vi "SA40144D.20210728 2D in vacuum.vi"() -> ()   [LabVIEW 2020]
uses:
  <vilib>/Analysis/baseanly.llb/Mean (DBL).vi
  <userlib>/_OpenG.lib/file/file.llb/Build Path - Traditional__ogtk.vi
  <userlib>/LevyLab/LV to ITX/Data/Data.lvclass
  <userlib>/LevyLab/XY Utilities/xy_utilities.lvlib
  <vilib>/Analysis/NI_AALBase.lvlib
panel:
  in  "Tab Control":enum32{"Page 1", "Page 2"}(tab)
  out "G2T vs t - X channel":T1(graph)
  out "G4T vs t - X channel":T1(graph)
  out "Temp vs t":T1(graph)
  out "Arrhenius":T1(graph)
  out "Y6 - dV":T1(graph)
  out "Y5 - I-":T1(graph)
  out "X5 - I-":T1(graph)
  out "X6 - dV":T1(graph)
  in  "Temps to keep (Lifespan)":i32=26
  out "E_a":dbl[](array[numeric])
  in  "Temps to keep (Arrhenius fit)":i32=26
  in  "Source Voltage":dbl=0.1
  in  "Init Temp":i32=275
  in  "Temp Step":i32=5
  in  "Final Temp":i32=400
  in  "Data File":path=path "G:/My Drive/ansom/Data/PPMS 2/SA40144D.20210728/00 - BG in vacuum/SA40144D.20210728.275K.dat"
  in  "Trimming":i32=400
  in  "Update":bool
  in  "OK":bool
  out "error out":errorcluster
  in  "error in (no error)":errorcluster
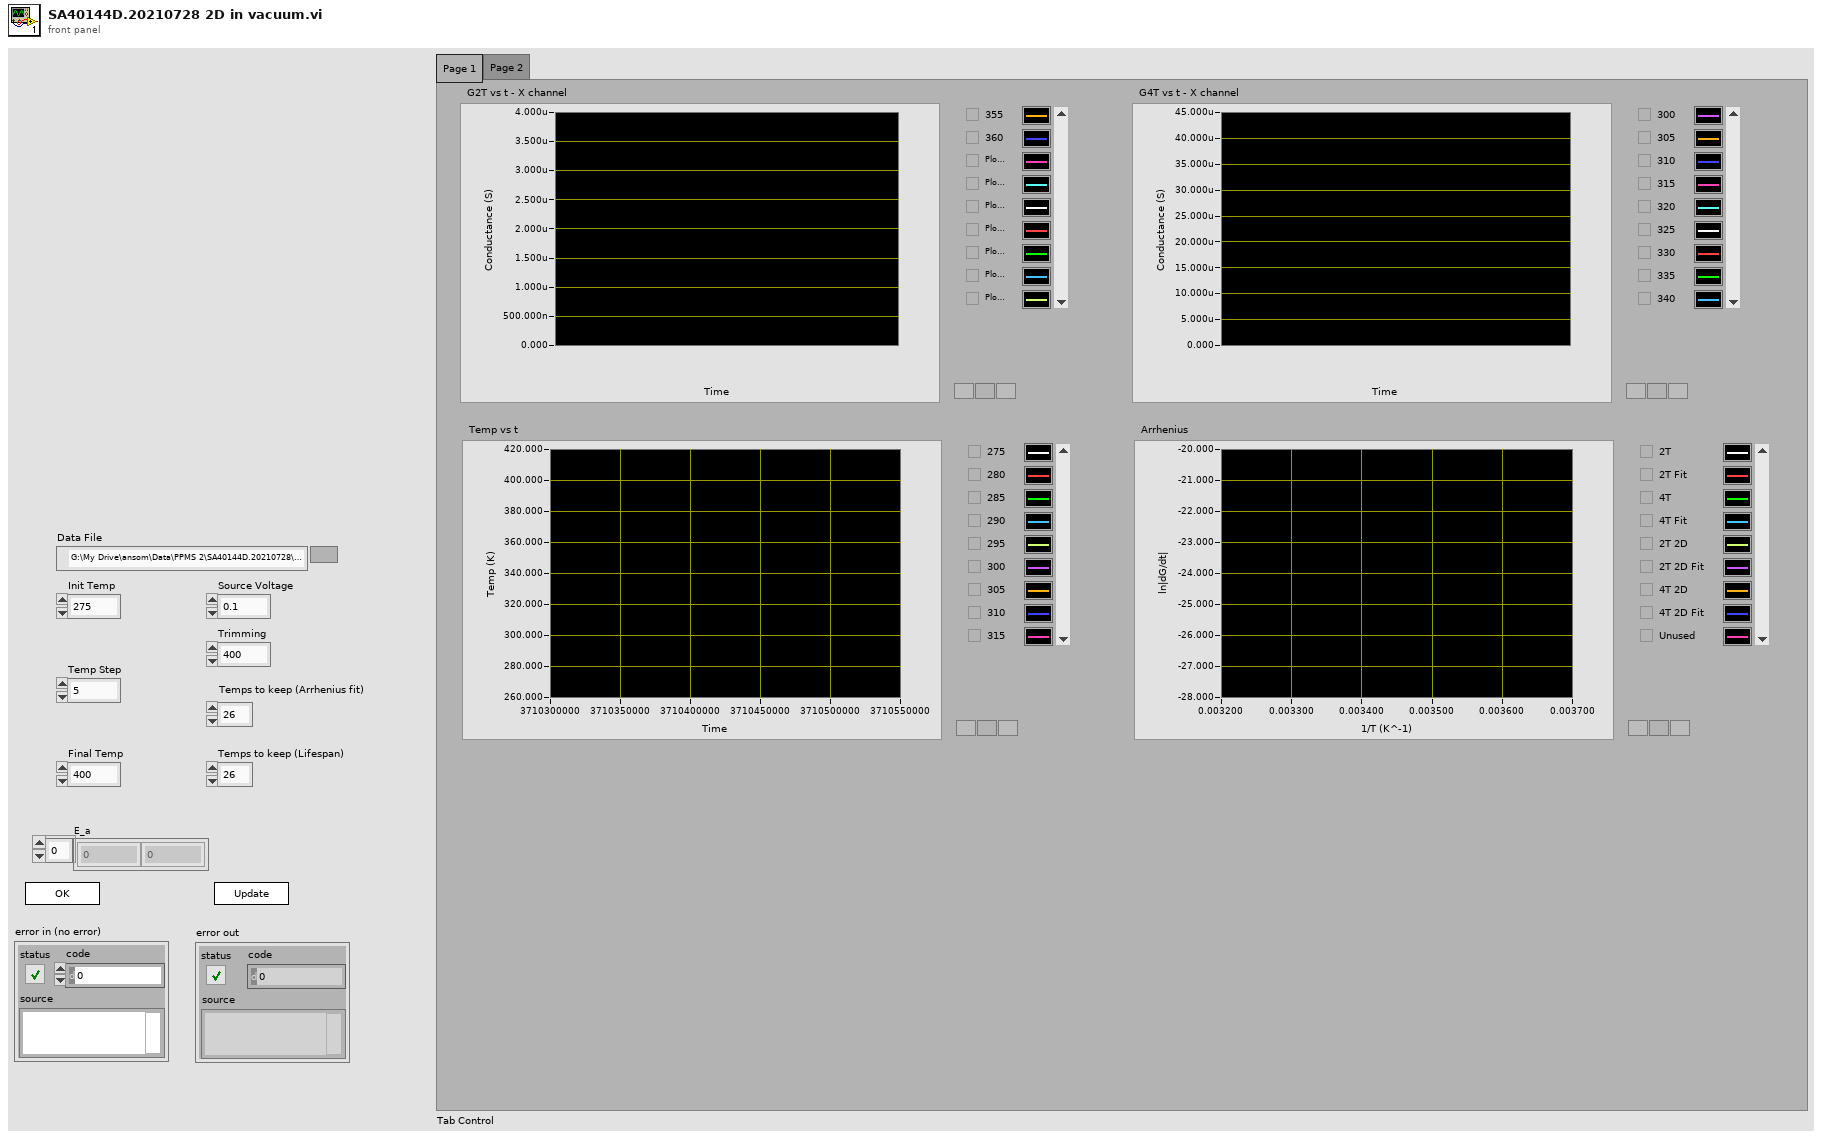
[diagram p1: front panel]
types:
  T1 = cluster{"Data":dbl[], "Best Exponential Fit":dbl[]}[]
  T2 = enum32{"Invalid", "Standard", "Closed", "Hidden", "Minimized", "Maximized"}
  T3 = enum32{"invalid app kind", "Development System", "Run Time System", "Student Edition", "Embedded LabVIEW", "Evaluation", "Custom"}
  T4 = cluster{"Core":cluster{"Current VI Reference":refnum<vi>, "Close Panel on Exit?":bool}, "G2T 1D":cluster{dbl[], dbl[]}[], "G4T 1D":cluster{dbl[], dbl[]}[], "X11":cluster{dbl[], dbl[]}[], "X15":cluster{dbl[], dbl[]}[], "Temp":cluster{dbl[], dbl[]}[], "G2T BG":cluster{dbl[], dbl[]}[], "Source Voltage":dbl, "Final Temp":i32, "Init Temp":i32, "Temp Step":i32, "Data File":path, "Trimming":i32}
  T5 = cluster{"Current VI Reference":refnum<vi>, "Close Panel on Exit?":bool}
  T6 = typedef "Data.lvclass/Dictionary--cluster.ctl" = cluster{"key":string, "value":variant}
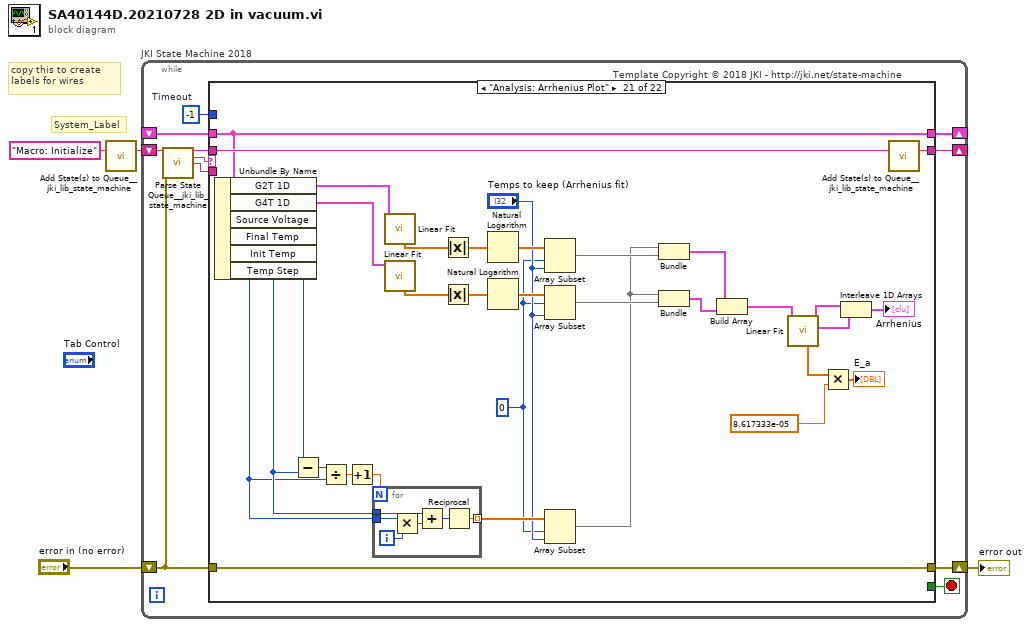
[diagram p0: block diagram]
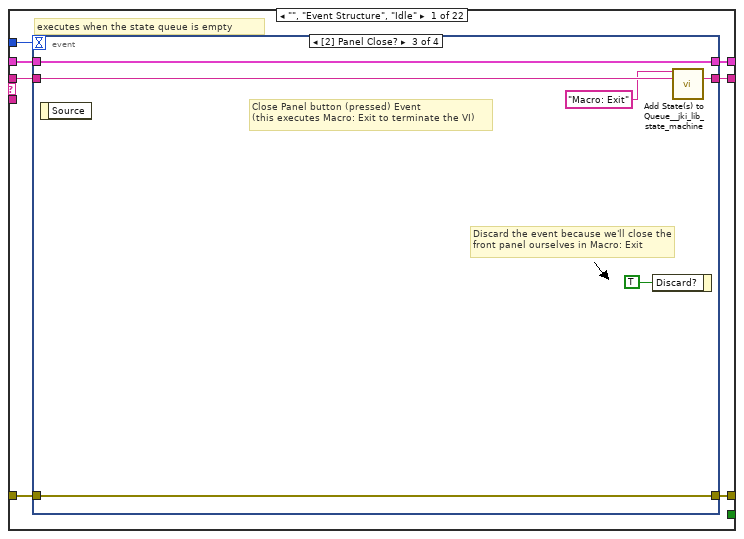
[diagram p2: hidden frame]
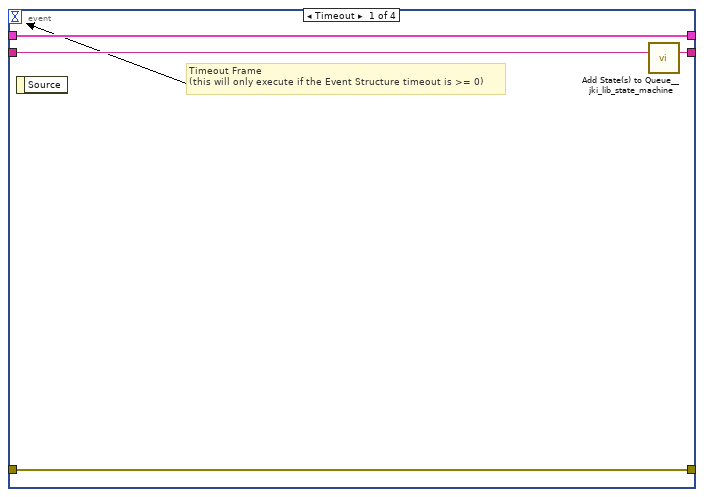
[diagram p3: hidden frame]
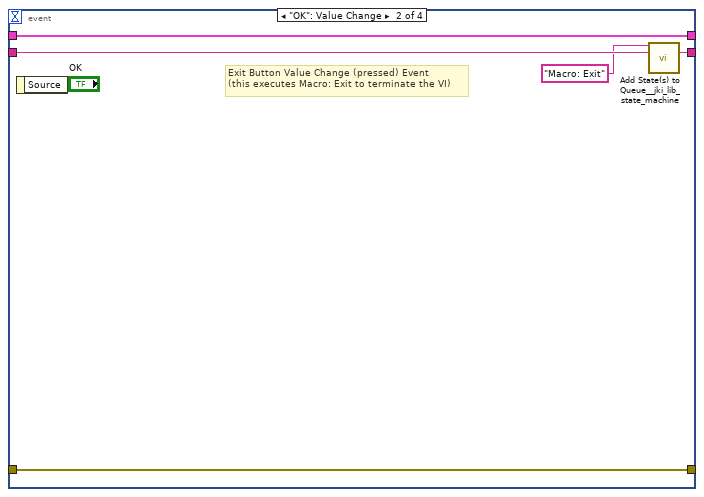
[diagram p4: hidden frame]
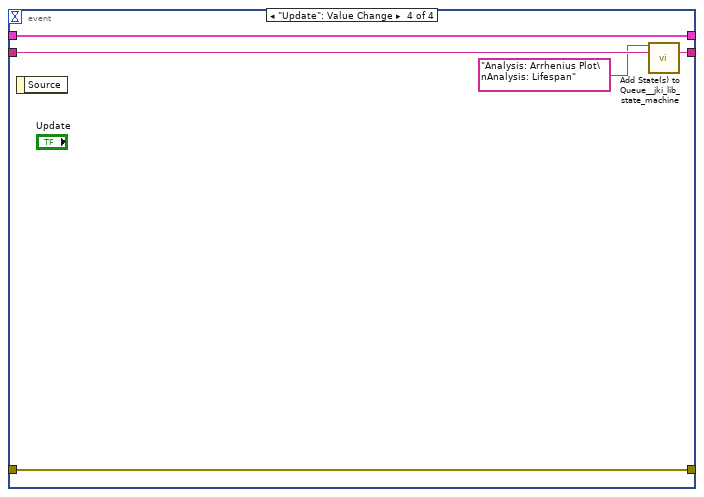
[diagram p5: hidden frame]
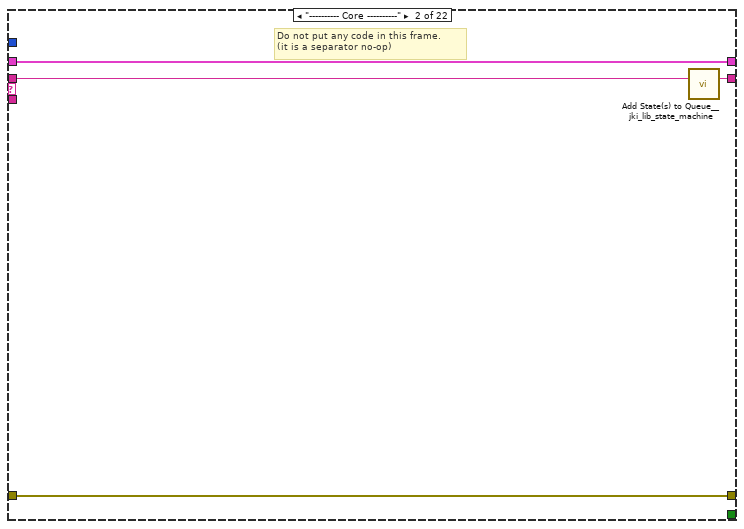
[diagram p6: hidden frame]
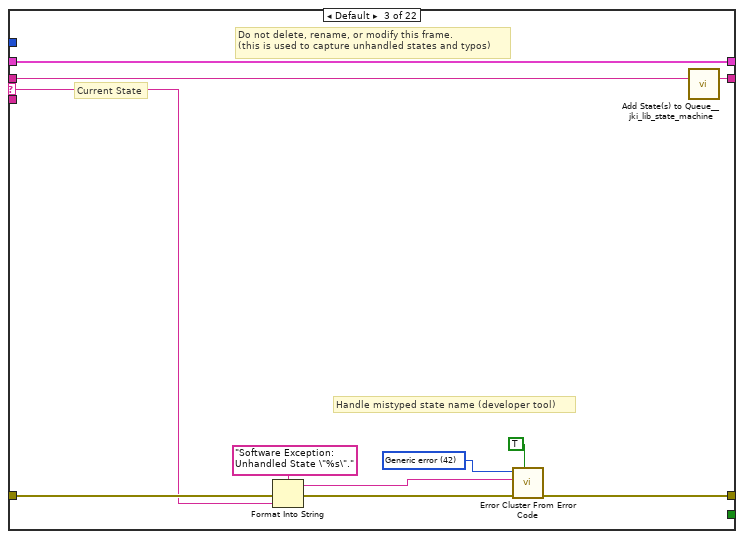
[diagram p7: hidden frame]
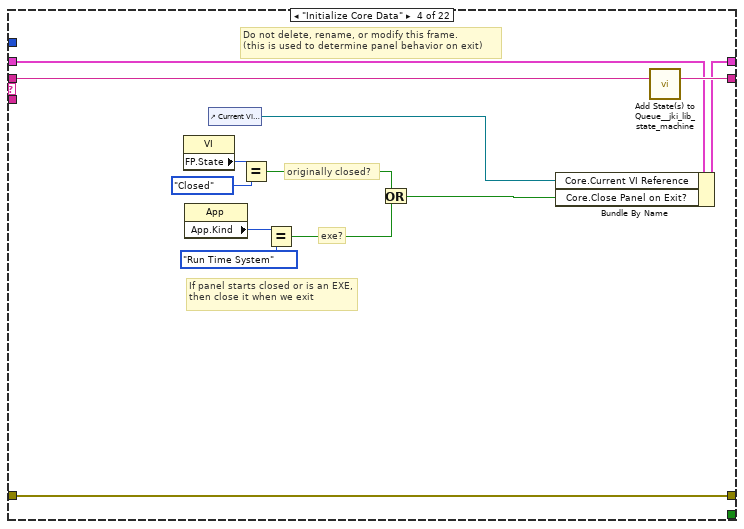
[diagram p8: hidden frame]
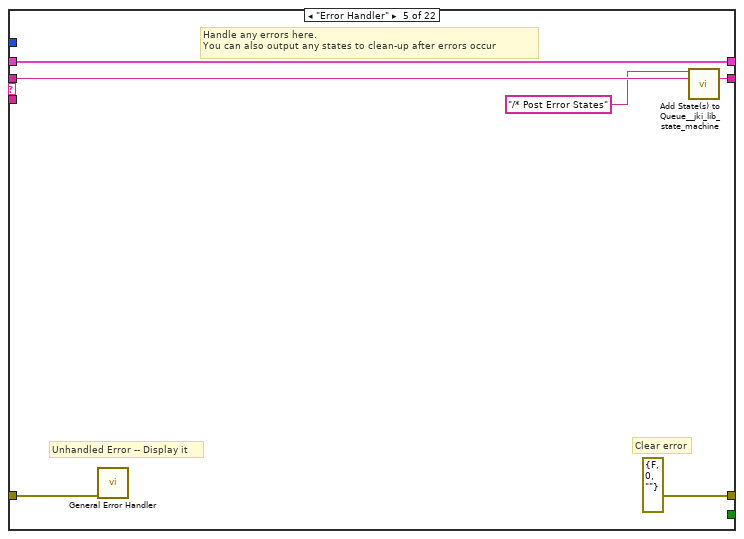
[diagram p9: hidden frame]
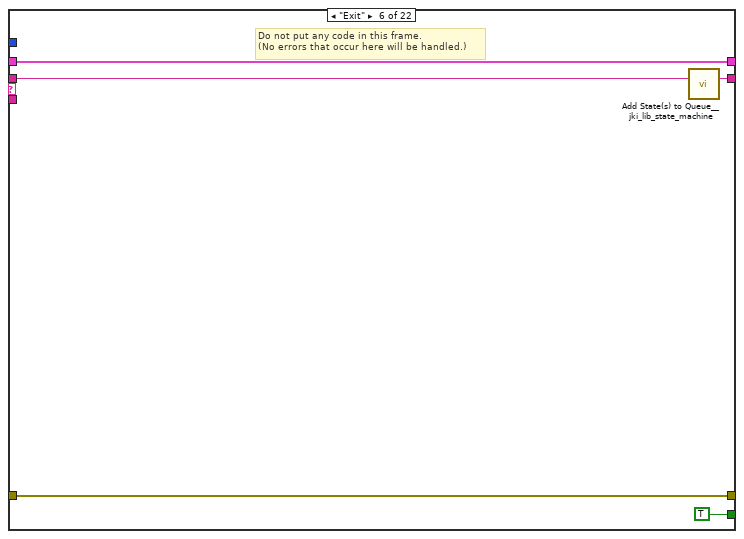
[diagram p10: hidden frame]
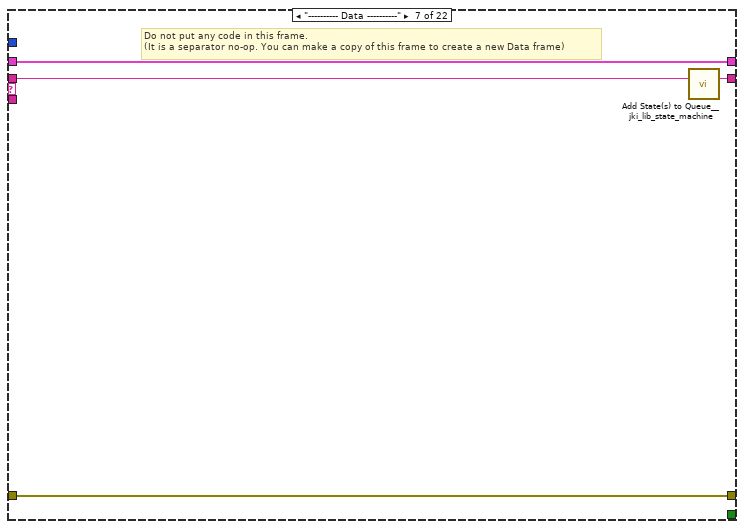
[diagram p11: hidden frame]
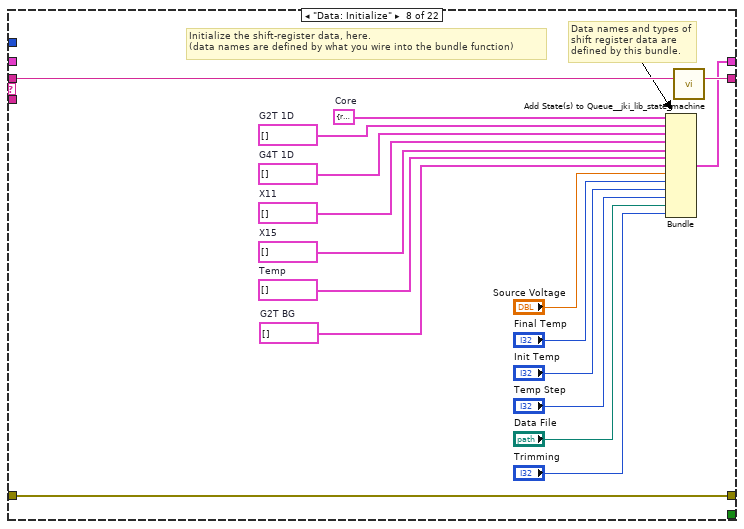
[diagram p12: hidden frame]
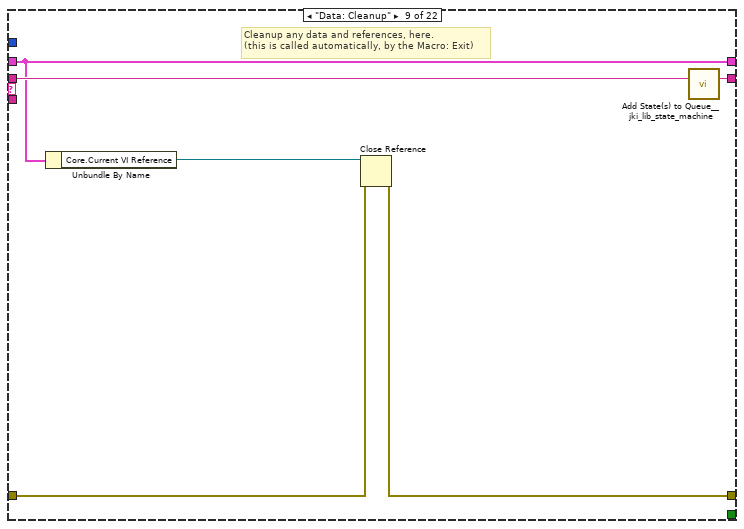
[diagram p13: hidden frame]
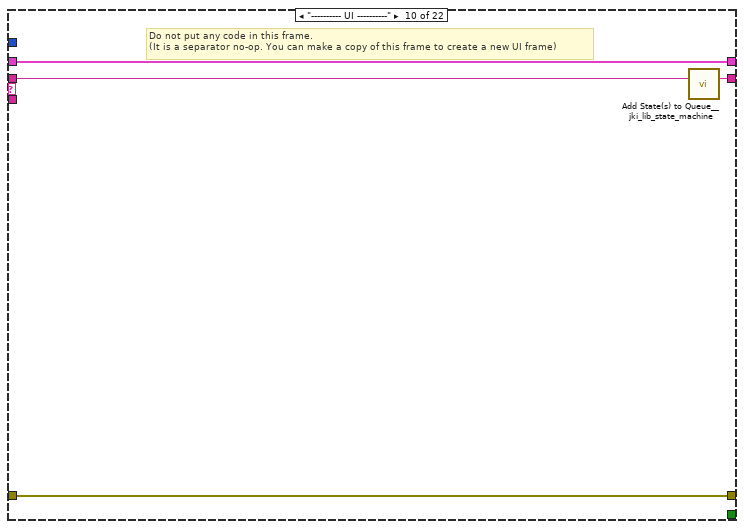
[diagram p14: hidden frame]
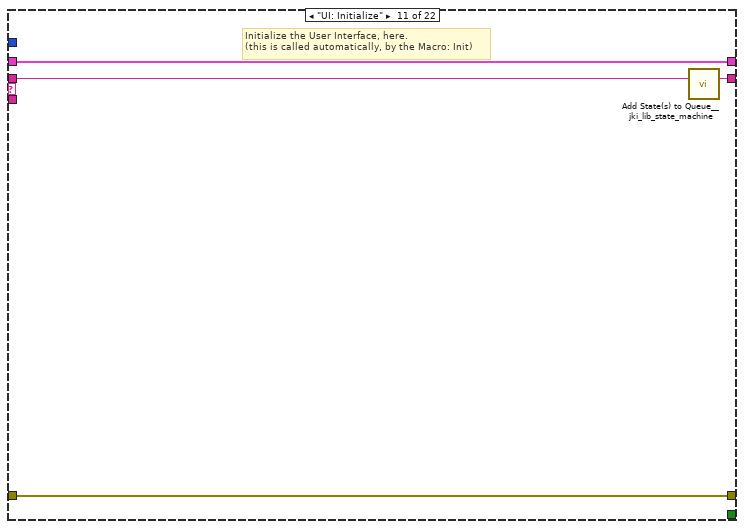
[diagram p15: hidden frame]
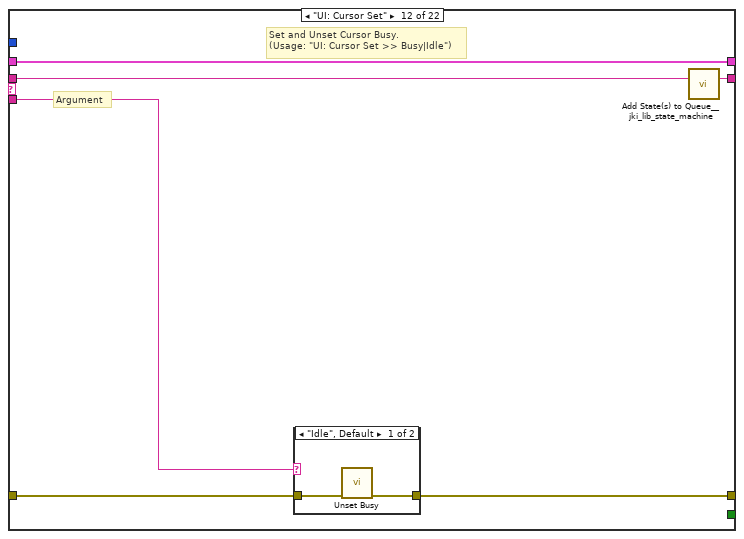
[diagram p16: hidden frame]
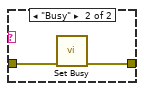
[diagram p17: hidden frame]
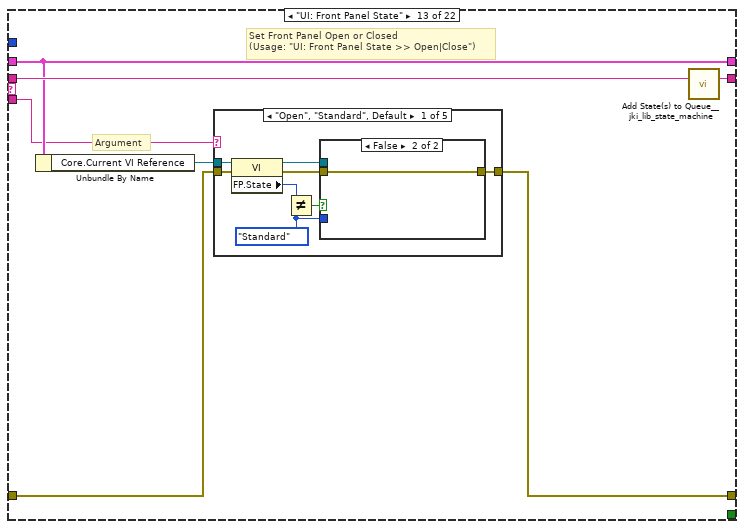
[diagram p18: hidden frame]
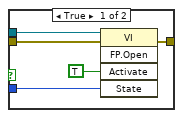
[diagram p19: hidden frame]
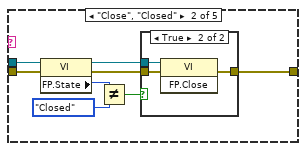
[diagram p20: hidden frame]
diagram:
  # "copy this to create labels for wires"
  # "System_Label"
  n1 = call <vilib>:"Add State(s) to Queue__jki_lib_state_machine.vi"("State(s) in (\"\")"="Macro: Initialize") -> ("States Out"=w4:string)  [unwired: 14 in]
  n2 = while "JKI State Machine 2018" {
    shift-right: [w8] -> _
    shift-left: _ -> [w7]
    shift-right: [w11] -> w1
    shift-left: "error in (no error)" -> [w5]
    shift-right: [w10] -> _
    shift-left: w4 -> [w12]
    stop <- w9 stop-if-true
    w6 = -1  # Timeout
    # "Template Copyright © 2018 JKI - http://jki.net/state-machine"
    n3 = call <vilib>:"Parse State Queue__jki_lib_state_machine.vi"("State Queue"=w12, "Error In (no error)"=w5) -> ("Remaining States"=w14:string, "Current State"=w15:string, "Arguments"=w13:string)  [unwired: 11 in]
    n4 = case shown="\"Analysis: Arrhenius Plot\"" w15 {
      selector: w15 -> [_ _ w47 _ _ _ _ _ _ _ _ _ _ _ _ _ _ _ _ _ _ _]
      tunnel: w14 -> [w22 w46 w51 w70 w76 w81 w85 w102 w108 w112 w116 w122 w133 w202 w207 w217 w221 w238 w295 w339 w372 w410]
      tunnel: w13 -> [_ _ _ _ _ _ _ _ _ _ _ w117 w127 _ _ _ _ _ _ _ _ _]
      tunnel: w7 -> [w20 w43 w49 w63 w73 w79 w82 _ w103 w109 w114 w120 w129 w199 w204 w214 w218 w232 w289 w336 w369 w396]
      tunnel: [w19 w44 w53 w67 errorcluster {"status"=FALSE, "code"=0, "source"=""} ("error out") w78 w83 w99 w104 w110 w113 w118 w130 w200 w205 w215 w219 w234 w291 w337 w370 w408] -> w11
      tunnel: w5 -> [w18 w44 w52 w67 w72 w78 w83 w99 w105 w110 w113 w119 w131 w200 w205 w215 w219 w234 w291 w337 w370 w408]
      tunnel: [w21 w45 w50 w69 w75 w80 w84 w101 w107 w111 w115 w121 w132 w201 w206 w216 w220 w237 w294 w338 w371 w409] -> w10
      tunnel: [_ _ _ _ _ TRUE _ _ _ _ _ _ _ _ _ _ _ _ _ _ _ _] -> w9
      tunnel: [w17 w43 w49 w68 w73 w79 w82 w100 w103 w109 w114 w120 w129 w199 w204 w214 w218 w233 w290 w336 w369 w396] -> w8
      tunnel: w6 -> [w16 _ _ _ _ _ _ _ _ _ _ _ _ _ _ _ _ _ _ _ _ _]
      frame "", "Event Structure", "Idle" {
        # "executes when the state queue is empty"
        n5 = event shown="[2] Panel Close?" {
          selector: _ -> [_ _ _ _]
          dyn-events: _ -> [_ _ _ _]
          timeout: w16 -> [_ _ _ _]
          tunnel: w22 -> [w26 w31 w37 w41]
          tunnel: [w25 w30 w36 w40] -> w21
          tunnel: w20 -> [w23 w28 w34 w42]
          tunnel: [w24 w29 w35 w38] -> w19
          tunnel: w18 -> [w24 w29 w35 w38]
          tunnel: [w23 w28 w34 w42] -> w17
          event Timeout {
            # "Timeout Frame\n(this will only execute if the Event Structure timeout is >= 0)"
            n6 = event-data() -> ()  [unwired: 1 in, 1 out]
            n7 = call <vilib>:"Add State(s) to Queue__jki_lib_state_machine.vi"("State(s) in (\"\")"=w26) -> ("States Out"=w25:string)  [unwired: 14 in]
          }
          event "OK": Value Change {
            # "Exit Button Value Change (pressed) Event\n(this executes Macro: Exit to terminate the VI)"
            n8 = event-data() -> ()  [unwired: 1 in, 1 out]
            n9 = call <vilib>:"Add State(s) to Queue__jki_lib_state_machine.vi"("State(s) in Front (\"\")"="Macro: Exit", "State(s) in (\"\")"=w31) -> ("States Out"=w30:string)  [unwired: 13 in]
          }
          event Panel Close? {
            # "Discard the event because we'll close the front panel ourselves in Macro: Exit"
            # "Close Panel button (pressed) Event\n(this executes Macro: Exit to terminate the VI)"
            n10 = event-data() -> ()  [unwired: 1 in, 1 out]
            n11 = event-data("Discard?"=TRUE) -> ()  [unwired: 1 in, 1 out]
            n12 = call <vilib>:"Add State(s) to Queue__jki_lib_state_machine.vi"("State(s) in Front (\"\")"="Macro: Exit", "State(s) in (\"\")"=w37) -> ("States Out"=w36:string)  [unwired: 13 in]
          }
          event "Update": Value Change {
            n13 = event-data() -> ()  [unwired: 1 in, 1 out]
            n14 = call <vilib>:"Add State(s) to Queue__jki_lib_state_machine.vi"("State(s) in Front (\"\")"="Analysis: Arrhenius Plot\nAnalysis: Lifespan" ("State(s) in Front (\"\")"), "State(s) in (\"\")"=w41) -> ("States Out"=w40:string)  [unwired: 13 in]
          }
        }
      }
      frame "---------- Core ----------" {
        # "Do not put any code in this frame.\n(it is a separator no-op)"
        n15 = call <vilib>:"Add State(s) to Queue__jki_lib_state_machine.vi"("State(s) in (\"\")"=w46) -> ("States Out"=w45:string)  [unwired: 14 in]
      }
      frame Default {
        w56 = 42 items=["No error", "Argument error", "Memory is full", "Out of zone", "End of file", "File already open", "Generic file I/O error", "File not found", "File permission error", "Disk is full", "Duplicate path", "Too many files open", "System feature not enabled", "Resource file not found", "Cannot add resource", "Resource not found", "Image not found", "Image memory error", "Pen does not exist", "Config type invalid", "Config token not found", "Config parse error", "Config memory error", "Bad external code format", "Bad external code offset", "External code not present", "Null window", "Destroy window error", "Null menu", "Print aborted", "Bad print record", "Print driver error", "Windows error during printing", "Memory error during printing", "Print dialog error", "Generic print error", "Invalid device refnum", "Device not found", "Device parameter error", "Device unit error", "Cannot open device", "Device call aborted", "Generic error", "Cancelled by user", "Object ID too low", "Object ID too high", "Object not in heap", "Unknown heap", "Unknown object (invalid DefProc)", "Unknown object (DefProc not in table)", "Message out of range", "Invalid (null) method", "Unknown message", "Manager call not supported", "Bad address", "Network operation in progress", "Network operation timed out", "Connection is busy", "Network attribute not supported", "Network error", "Address in use", "System out of memory", "Connection aborted", "Connection refused", "Not connected", "Already connected", "Connection closed", "Initialization error (interapplication manager)", "Bad occurrence", "Wait on unbound occurrence handler", "Occurrence queue overflow", "Datalog type conflict", "Unused", "Unrecognized type (interapplication manager)", "Memory corrupt", "Failed to make temporary DLL", "Old CIN version", "Drag socket not found", "Failed to load drop-object", "Failed to register OLE object", "Failed to release OLE object", "Format specifier type mismatch", "Unknown format specifier", "Too few format specifiers", "Too many format specifiers", "Scan failed", "Newer CIN version", "Error converting to variant", "Runtime menu error", "Password tampered", "Variant attribute not found", "Incompatible variant data type", "Event data is not available", "Event Store is not present", "Occurrence is not found", "Event Queue is not created", "Event info is not available", "Refnum passed is NULL", "Error retrieving Class GUID", "Error retrieving CoClass GUID", "Error retrieving TypeLib GUID.", "Bad built application magic bytes.", "Specific driver is different from the specific driver associated with the Logical Name.", "There is no session opened to the class driver.", "Max Error", "MAX - Error with config objects", "MAX - Error loading configuration", "MAX - Group not supported"]
        # "Current State"
        # "Do not delete, rename, or modify this frame.\n(this is used to capture unhandled states and typos)"
        # "Handle mistyped state name (developer tool)"
        n16 = Format Into String(format string="Software Exception: Unhandled State \"%s\"." ("message"), error in=w52, w47) -> (resulting string=w55:string, error out=w54:errorcluster)  [unwired: 1 in]
        n17 = call <vilib>:"Error Cluster From Error Code.vi"("show call chain? (False)"=TRUE, "error in (no error)"=w54, "error message (\"\")"=w55, "error code (0)"=w56) -> ("error out"=w53:errorcluster)  [unwired: 5 in]
        n18 = call <vilib>:"Add State(s) to Queue__jki_lib_state_machine.vi"("State(s) in (\"\")"=w51) -> ("States Out"=w50:string)  [unwired: 14 in]
      }
      frame "Initialize Core Data" {
        # "Do not delete, rename, or modify this frame.\n(this is used to determine panel behavior on exit)"
        # "originally closed?"
        # "exe?"
        # "If panel starts closed or is an EXE, then close it when we exit"
        n19 = property class="VI"() -> ("FP.State"=w60:T2)  [unwired: 2 in, 2 out]
        n20 = property class="App"() -> ("App.Kind"=w66:T3)  [unwired: 2 in, 2 out]
        n21 = control-ref of="Current VI Reference"() -> (w61:refnum<vi>)
        n22 = Equal?(x=w60, y=T2."Closed" ("Front Panel Window:State")) -> (x = y?=w58:bool)
        n23 = Equal?(x=w66, y=T3."Run Time System" ("Application:Kind")) -> (x = y?=w64:bool)
        n24 = Or(x=w58, y=w64) -> (x .or. y?=w62:bool)
        n25 = Bundle By Name(cluster=w63, "Core.Current VI Reference"=w61, "Core.Close Panel on Exit?"=w62) -> (w68:T4)
        n26 = call <vilib>:"Add State(s) to Queue__jki_lib_state_machine.vi"("State(s) in (\"\")"=w70) -> ("States Out"=w69:string)  [unwired: 14 in]
      }
      frame "Error Handler" {
        # "Unhandled Error -- Display it"
        # "Handle any errors here.\nYou can also output any states to clean-up after errors occur"
        # "Clear error"
        n27 = call <vilib>:"General Error Handler.vi"("error in (no error)"=w72) -> ()  [unwired: 10 in, 5 out]
        n28 = call <vilib>:"Add State(s) to Queue__jki_lib_state_machine.vi"("State(s) in Front (\"\")"="/* Post Error States", "State(s) in (\"\")"=w76) -> ("States Out"=w75:string)  [unwired: 13 in]
      }
      frame "Exit" {
        # "Do not put any code in this frame.\n(No errors that occur here will be handled.)"
        n29 = call <vilib>:"Add State(s) to Queue__jki_lib_state_machine.vi"("State(s) in (\"\")"=w81) -> ("States Out"=w80:string)  [unwired: 14 in]
      }
      frame "---------- Data ----------" {
        # "Do not put any code in this frame.\n(It is a separator no-op. You can make a copy of this frame to create a new Data frame)"
        n30 = call <vilib>:"Add State(s) to Queue__jki_lib_state_machine.vi"("State(s) in (\"\")"=w85) -> ("States Out"=w84:string)  [unwired: 14 in]
      }
      frame "Data: Initialize" {
        w86 = cluster{dbl[], dbl[]}[] []  # G2T BG
        w87 = cluster{dbl[], dbl[]}[] []  # Temp
        w96 = cluster{dbl[], dbl[]}[] []  # X15
        w95 = cluster{dbl[], dbl[]}[] []  # X11
        w94 = cluster{dbl[], dbl[]}[] []  # G4T 1D
        w93 = cluster{dbl[], dbl[]}[] []  # G2T 1D
        w98 = T5 {"Current VI Reference"=refnum, "Close Panel on Exit?"=FALSE}  # Core
        # "Data names and types of shift register data are defined by this bundle."
        # "Initialize the shift-register data, here.\n(data names are defined by what you wire into the bundle function)"
        n31 = Bundle("Core"=w98, "G2T 1D"=w93, "G4T 1D"=w94, "X11"=w95, "X15"=w96, "Temp"=w87, "G2T BG"=w86, "Source Voltage"="Source Voltage", "Final Temp"="Final Temp", "Init Temp"="Init Temp", "Temp Step"="Temp Step", "Data File"="Data File", "Trimming"="Trimming") -> (w100:T4)  [unwired: 1 in]
        n32 = call <vilib>:"Add State(s) to Queue__jki_lib_state_machine.vi"("State(s) in (\"\")"=w102) -> ("States Out"=w101:string)  [unwired: 14 in]
      }
      frame "Data: Cleanup" {
        # "Cleanup any data and references, here.\n(this is called automatically, by the Macro: Exit)"
        n33 = Unbundle By Name(w103) -> ("Core.Current VI Reference"=w106:refnum<vi>)
        n34 = Close Reference(reference=w106, error in (no error)=w105) -> (error out=w104:errorcluster)
        n35 = call <vilib>:"Add State(s) to Queue__jki_lib_state_machine.vi"("State(s) in (\"\")"=w108) -> ("States Out"=w107:string)  [unwired: 14 in]
      }
      frame "---------- UI ----------" {
        # "Do not put any code in this frame.\n(It is a separator no-op. You can make a copy of this frame to create a new UI frame)"
        n36 = call <vilib>:"Add State(s) to Queue__jki_lib_state_machine.vi"("State(s) in (\"\")"=w112) -> ("States Out"=w111:string)  [unwired: 14 in]
      }
      frame "UI: Initialize" {
        # "Initialize the User Interface, here.\n(this is called automatically, by the Macro: Init)"
        n37 = call <vilib>:"Add State(s) to Queue__jki_lib_state_machine.vi"("State(s) in (\"\")"=w116) -> ("States Out"=w115:string)  [unwired: 14 in]
      }
      frame "UI: Cursor Set" {
        # "Argument"
        # "Set and Unset Cursor Busy.\n(Usage: \"UI: Cursor Set >> Busy|Idle\")"
        n38 = case shown="\"Idle\", Default" w117 {
          tunnel: w119 -> [w124 w126]
          tunnel: [w123 w125] -> w118
          frame "Idle", Default {
            n39 = call <vilib>:"Unset Busy.vi"("error in (no error)"=w124) -> ("error out"=w123:errorcluster)  [unwired: 10 in]
          }
          frame "Busy" {
            n40 = call <vilib>:"Set Busy.vi"("error in (no error)"=w126) -> ("error out"=w125:errorcluster)  [unwired: 9 in, 1 out]
          }
        }
        n41 = call <vilib>:"Add State(s) to Queue__jki_lib_state_machine.vi"("State(s) in (\"\")"=w122) -> ("States Out"=w121:string)  [unwired: 14 in]
      }
      frame "UI: Front Panel State" {
        # "Argument"
        # "Set Front Panel Open or Closed\n(Usage: \"UI: Front Panel State >> Open|Close\")"
        n42 = Unbundle By Name(w129) -> ("Core.Current VI Reference"=w128:refnum<vi>)
        n43 = case shown="\"Open\", \"Standard\", Default" w127 {
          tunnel: w131 -> [w139 w154 w165 w178 w191]
          tunnel: [w141 w155 w167 w180 w193] -> w130
          tunnel: w128 -> [w140 w152 w166 w179 w192]
          frame "Open", "Standard", Default {
            w134 = T2."Standard" ("State")
            n44 = property class="VI"(reference=w140, error in=w139) -> (reference out=w137:refnum<vi>, error out=w138:errorcluster, "FP.State"=w136:T2)
            n45 = Not Equal?(x=w136, y=w134) -> (x != y?=w135:bool)
            n46 = case shown="False" w135 {
              tunnel: [w145 w147] -> w141
              tunnel: w138 -> [w144 w147]
              tunnel: w137 -> [w143 _]
              tunnel: w134 -> [w142 _]
              frame True {
                n47 = invoke class="VI" method="FP.Open"(reference=w143, error in=w144, "Activate"=TRUE, "State"=w142) -> (error out=w145:errorcluster)  [unwired: 1 in, 4 out]
              }
              frame False {
              }
            }
          }
          frame "Close", "Closed" {
            n48 = property class="VI"(reference=w152, error in=w154) -> (reference out=w151:refnum<vi>, error out=w153:errorcluster, "FP.State"=w149:T2)
            n49 = Not Equal?(x=w149, y=T2."Closed" ("Front Panel Window:State")) -> (x != y?=w148:bool)
            n50 = case shown="True" w148 {
              tunnel: [w156 w159] -> w155
              tunnel: w153 -> [w156 w158]
              tunnel: w151 -> [_ w157]
              frame False {
              }
              frame True {
                n51 = invoke class="VI" method="FP.Close"(reference=w157, error in=w158) -> (error out=w159:errorcluster)  [unwired: 1 in, 2 out]
              }
            }
          }
          frame "Hidden", "Hide" {
            w160 = T2."Hidden" ("State")
            n52 = property class="VI"(reference=w166, error in=w165) -> (reference out=w163:refnum<vi>, error out=w164:errorcluster, "FP.State"=w162:T2)
            n53 = Not Equal?(x=w162, y=w160) -> (x != y?=w161:bool)
            n54 = case shown="True" w161 {
              tunnel: [w171 w172] -> w167
              tunnel: w164 -> [w170 w172]
              tunnel: w163 -> [w169 _]
              tunnel: w160 -> [w168 _]
              frame True {
                n55 = invoke class="VI" method="FP.Open"(reference=w169, error in=w170, "State"=w168) -> (error out=w171:errorcluster)  [unwired: 2 in, 4 out]
              }
              frame False {
              }
            }
          }
          frame "Minimize", "Minimized" {
            w173 = T2."Minimized" ("State")
            n56 = property class="VI"(reference=w179, error in=w178) -> (reference out=w176:refnum<vi>, error out=w177:errorcluster, "FP.State"=w175:T2)
            n57 = Not Equal?(x=w175, y=w173) -> (x != y?=w174:bool)
            n58 = case shown="True" w174 {
              tunnel: [w184 w185] -> w180
              tunnel: w177 -> [w183 w185]
              tunnel: w176 -> [w182 _]
              tunnel: w173 -> [w181 _]
              frame True {
                n59 = invoke class="VI" method="FP.Open"(reference=w182, error in=w183, "State"=w181) -> (error out=w184:errorcluster)  [unwired: 2 in, 4 out]
              }
              frame False {
              }
            }
          }
          frame "Maximize", "Maximized" {
            w186 = T2."Maximized" ("State")
            n60 = property class="VI"(reference=w192, error in=w191) -> (reference out=w189:refnum<vi>, error out=w190:errorcluster, "FP.State"=w188:T2)
            n61 = Not Equal?(x=w188, y=w186) -> (x != y?=w187:bool)
            n62 = case shown="True" w187 {
              tunnel: [w197 w198] -> w193
              tunnel: w190 -> [w196 w198]
              tunnel: w189 -> [w195 _]
              tunnel: w186 -> [w194 _]
              frame True {
                n63 = invoke class="VI" method="FP.Open"(reference=w195, error in=w196, "State"=w194) -> (error out=w197:errorcluster)  [unwired: 2 in, 4 out]
              }
              frame False {
              }
            }
          }
        }
        n64 = call <vilib>:"Add State(s) to Queue__jki_lib_state_machine.vi"("State(s) in (\"\")"=w133) -> ("States Out"=w132:string)  [unwired: 14 in]
      }
      frame "---------- Macro ----------" {
        # "Do not put any code in this frame.\n(It is a separator no-op. You can make a copy of this frame to create a new Macro frame)"
        n65 = call <vilib>:"Add State(s) to Queue__jki_lib_state_machine.vi"("State(s) in (\"\")"=w202) -> ("States Out"=w201:string)  [unwired: 14 in]
      }
      frame "Macro: Initialize" {
        # "Initialization Macro\n(This is called once, when the VI starts)"
        n66 = call <vilib>:"Add State(s) to Queue__jki_lib_state_machine.vi"("State(s) in Front (\"\")"="Data: Initialize\nInitialize Core Data\nUI: Initialize\nUI: Front Panel State >> Open\nAnalysis: Load 1D\nAnalysis: Load X\nAnalysis: Plot G vs t\nAnalysis: Arrhenius Plot\nAnalysis: Lifespan", "State(s) in (\"\")"=w207) -> ("States Out"=w206:string)  [unwired: 13 in]
      }
      frame "Macro: Exit" {
        # "Exit Macro\n(This is called once, when the VI exits)"
        n67 = Unbundle By Name(w214) -> ("Core.Close Panel on Exit?"=w213:bool)
        n68 = Select(t="UI: Front Panel State >> Close", s=w213, f="") -> (s? t:f=w210:string)
        n69 = call <vilib>:"Add State(s) to Queue__jki_lib_state_machine.vi"("State(s) in (\"\")"=w210, "State(s) at Back (\"\")"="Data: Cleanup\nExit") -> ("States Out"=w208:string)  [unwired: 13 in]
        n70 = call <vilib>:"Add State(s) to Queue__jki_lib_state_machine.vi"("State(s) in Front (\"\")"=w208, "State(s) in (\"\")"=w217) -> ("States Out"=w216:string)  [unwired: 13 in]
      }
      frame "---------- Analysis ----------" {
        # "Template Separator\n(You can make a copy of, or modify, this frame)"
        n71 = call <vilib>:"Add State(s) to Queue__jki_lib_state_machine.vi"("State(s) in (\"\")"=w221) -> ("States Out"=w220:string)  [unwired: 14 in]
      }
      frame "Analysis: Load 1D" {
        n72 = Unbundle By Name(w232) -> ("Source Voltage"=w231:dbl, "Final Temp"=w228:i32, "Init Temp"=w225:i32, "Temp Step"=w224:i32, "Data File"=w226:path, "Trimming"=w223:i32)
        n73 = Subtract(x=w228, y=w225) -> (x-y=w235:i32)
        n74 = Divide(x=w235, y=w224) -> (x/y=w236:dbl)
        n75 = Increment(x=w236) -> (x+1=w227:dbl)
        n76 = for {
          N: w227 -> [_]
          tunnel: w231 -> [w243]
          tunnel: [w266] -> w230 mode=indexing
          tunnel: [w265] -> w229 mode=indexing
          tunnel: w226 -> [w264]
          tunnel: w225 -> [w263]
          tunnel: w224 -> [w262]
          tunnel: w223 -> [w245]
          tunnel: [w260] -> w222 mode=indexing
          i -> [w269]
          n77 = Strip Path(path=w264) -> (stripped path=w274:path, name=w273:string)
          n78 = Multiply(x=w262, y=w269) -> (x*y=w270:i32)
          n79 = Add(x=w263, y=w270) -> (x+y=w275:i32)
          n80 = String Subset(string=w273, length (rest)=18) -> (substring=w271:string)  [unwired: 1 in]
          n81 = Format Into String(w275) -> (resulting string=w277:string)  [unwired: 3 in, 1 out]
          n82 = Concatenate Strings(w271, w277, "K.dat" ("string")) -> (w276:string)
          n83 = call-poly <userlib>:"Build Path__ogtk.vi"("name or relative path"=w276, "base path"=w274) -> ("appended path"=w278:path)
          n84 = call <userlib>:"Data Read.vi"("path"=w278) -> ("Data (Dictionary)"=w247:T6[])  [unwired: 7 in, 3 out]
          n85 = call "Read Dictionary.vi"("Numeric"=0, "Dictionary In"=w247) -> ("data"=w256:dbl[])
          n86 = call "Read Dictionary.vi"("Numeric"=7 ("index"), "Dictionary In"=w247) -> ("data"=w252:dbl[])
          n87 = call "Read Dictionary.vi"("Numeric"=6 ("index"), "Dictionary In"=w247) -> ("data"=w246:dbl[])
          n88 = call "Read Dictionary.vi"("Numeric"=5, "Dictionary In"=w247) -> ("data"=w255:dbl[])
          n89 = call "Read Dictionary.vi"("Numeric"=1, "Dictionary In"=w247) -> ("data"=w254:dbl[])
          n90 = Array Subset(array=w256, index=w245) -> (w242:dbl[])  [unwired: 1 in]
          n91 = Array Subset(array=w252, index=w245) -> (w244:dbl[])  [unwired: 1 in]
          n92 = Array Subset(array=w246, index=w245) -> (w241:dbl[])  [unwired: 1 in]
          n93 = Array Subset(array=w255, index=w245) -> (w240:dbl[])  [unwired: 1 in]
          n94 = Subtract(x=w241, y=w240) -> (x-y=w239:dbl[])
          n95 = Divide(x=w244, y=w243) -> (x/y=w268:dbl[])
          n96 = Array Subset(array=w254) -> (w261:dbl[])  [unwired: 2 in]
          n97 = Absolute Value(x=w268) -> (abs(x)=w251:dbl[])
          n98 = Divide(x=w244, y=w239) -> (x/y=w249:dbl[])
          n99 = Bundle(w242, w251) -> (w266:cluster{dbl[], dbl[]})  [unwired: 1 in]
          n100 = Bundle(w242, w261) -> (w260:cluster{dbl[], dbl[]})  [unwired: 1 in]
          n101 = Absolute Value(x=w249) -> (abs(x)=w250:dbl[])
          n102 = Bundle(w242, w250) -> (w265:cluster{dbl[], dbl[]})  [unwired: 1 in]
        }
        n103 = call <vilib>:"Add State(s) to Queue__jki_lib_state_machine.vi"("State(s) in (\"\")"=w238) -> ("States Out"=w237:string)  [unwired: 14 in]
        n104 = Bundle By Name(cluster=w232, "G2T 1D"=w230, "G4T 1D"=w229, "Temp"=w222) -> (w233:T4)
      }
      frame "Analysis: Load X" {
        n105 = Unbundle By Name(w289) -> ("Final Temp"=w287:i32, "Init Temp"=w284:i32, "Temp Step"=w283:i32, "Data File"=w285:path, "Trimming"=w282:i32)  [unwired: 1 out]
        n106 = Subtract(x=w287, y=w284) -> (x-y=w292:i32)
        n107 = Divide(x=w292, y=w283) -> (x/y=w293:dbl)
        n108 = Increment(x=w293) -> (x+1=w286:dbl)
        n109 = for {
          N: w286 -> [_]
          tunnel: [w319] -> w281 mode=indexing
          tunnel: [w318] -> w288 mode=indexing
          tunnel: w285 -> [w317]
          tunnel: w284 -> [w316]
          tunnel: w283 -> [w315]
          tunnel: w282 -> [w301]
          tunnel: [w297] -> w280 mode=indexing
          tunnel: [w296] -> w279 mode=indexing
          i -> [w321]
          n110 = Strip Path(path=w317) -> (stripped path=w326:path, name=w325:string)
          n111 = Multiply(x=w315, y=w321) -> (x*y=w322:i32)
          n112 = Add(x=w316, y=w322) -> (x+y=w327:i32)
          n113 = String Subset(string=w325, length (rest)=18) -> (substring=w323:string)  [unwired: 1 in]
          n114 = Format Into String(w327) -> (resulting string=w329:string)  [unwired: 3 in, 1 out]
          n115 = Concatenate Strings(w323, w329, "K.dat" ("string")) -> (w328:string)
          n116 = call-poly <userlib>:"Build Path__ogtk.vi"("name or relative path"=w328, "base path"=w326) -> ("appended path"=w330:path)
          n117 = call <userlib>:"Data Read.vi"("path"=w330) -> ("Data (Dictionary)"=w306:T6[])  [unwired: 7 in, 3 out]
          n118 = call "Read Dictionary.vi"("Numeric"=0, "Dictionary In"=w306) -> ("data"=w312:dbl[])
          n119 = call "Read Dictionary.vi"("Numeric"=7 ("index"), "Dictionary In"=w306) -> ("data"=w309:dbl[])
          n120 = call "Read Dictionary.vi"("Numeric"=8, "Dictionary In"=w306) -> ("data"=w311:dbl[])
          n121 = call "Read Dictionary.vi"("Numeric"=15, "Dictionary In"=w306) -> ("data"=w303:dbl[])
          n122 = call "Read Dictionary.vi"("Numeric"=16, "Dictionary In"=w306) -> ("data"=w302:dbl[])
          n123 = Array Subset(array=w312, index=w301) -> (w298:dbl[])  [unwired: 1 in]
          n124 = Array Subset(array=w309, index=w301) -> (w307:dbl[])  [unwired: 1 in]
          n125 = Array Subset(array=w311, index=w301) -> (w308:dbl[])  [unwired: 1 in]
          n126 = Array Subset(array=w303, index=w301) -> (w300:dbl[])  [unwired: 1 in]
          n127 = Array Subset(array=w302, index=w301) -> (w299:dbl[])  [unwired: 1 in]
          n128 = Bundle(w298, w300) -> (w297:cluster{dbl[], dbl[]})  [unwired: 1 in]
          n129 = Bundle(w298, w299) -> (w296:cluster{dbl[], dbl[]})  [unwired: 1 in]
          n130 = Bundle(w298, w307) -> (w319:cluster{dbl[], dbl[]})  [unwired: 1 in]
          n131 = Bundle(w298, w308) -> (w318:cluster{dbl[], dbl[]})  [unwired: 1 in]
        }
        "Y6 - dV" <- w279
        "Y5 - I-" <- w280
        n132 = call <vilib>:"Add State(s) to Queue__jki_lib_state_machine.vi"("State(s) in (\"\")"=w295) -> ("States Out"=w294:string)  [unwired: 14 in]
        n133 = Bundle By Name(cluster=w289, "X11"=w281, "X15"=w288) -> (w290:T4)
      }
      frame "Analysis: Plot G vs t" {
        n134 = Unbundle By Name(w336) -> ("G2T 1D"=→"G2T vs t - X channel":cluster{dbl[], dbl[]}[], "G4T 1D"=→"G4T vs t - X channel":cluster{dbl[], dbl[]}[], "X11"=→"X5 - I-":cluster{dbl[], dbl[]}[], "X15"=→"X6 - dV":cluster{dbl[], dbl[]}[], "Temp"=→"Temp vs t":cluster{dbl[], dbl[]}[])
        n135 = call <vilib>:"Add State(s) to Queue__jki_lib_state_machine.vi"("State(s) in (\"\")"=w339) -> ("States Out"=w338:string)  [unwired: 14 in]
      }
      frame "Analysis: Arrhenius Plot" {
        w340 = 0
        n136 = Unbundle By Name(w369) -> ("G2T 1D"=w344:cluster{dbl[], dbl[]}[], "G4T 1D"=w343:cluster{dbl[], dbl[]}[], "Final Temp"=w366:i32, "Init Temp"=w364:i32, "Temp Step"=w363:i32)  [unwired: 1 out]
        n137 = Subtract(x=w366, y=w364) -> (x-y=w367:i32)
        n138 = Divide(x=w367, y=w363) -> (x/y=w368:dbl)
        n139 = Increment(x=w368) -> (x+1=w365:dbl)
        n140 = for {
          N: w365 -> [_]
          tunnel: w364 -> [w375]
          tunnel: w363 -> [w376]
          tunnel: [w373] -> w355 mode=indexing
          i -> [w377]
          n141 = Multiply(x=w376, y=w377) -> (x*y=w378:i32)
          n142 = Add(x=w375, y=w378) -> (x+y=w374:i32)
          n143 = Reciprocal(x=w374) -> (1/x=w373:dbl)
        }
        n144 = call-poly <userlib>:"Linear Fit.vi"("XY-data"=w344) -> ("slopes"=w341:dbl[])  [unwired: 4 in, 6 out]
        n145 = call-poly <userlib>:"Linear Fit.vi"("XY-data"=w343) -> ("slopes"=w342:dbl[])  [unwired: 4 in, 6 out]
        n146 = Absolute Value(x=w341) -> (abs(x)=w361:dbl[])
        n147 = Absolute Value(x=w342) -> (abs(x)=w362:dbl[])
        n148 = Natural Logarithm(1:w361) -> (0:w357:dbl[])
        n149 = Natural Logarithm(1:w362) -> (0:w356:dbl[])
        n150 = Array Subset(array=w357, index=w340, length="Temps to keep (Arrhenius fit)") -> (w353:dbl[])
        n151 = Array Subset(array=w356, index=w340, length="Temps to keep (Arrhenius fit)") -> (w352:dbl[])
        n152 = Array Subset(array=w355, index=w340, length="Temps to keep (Arrhenius fit)") -> (w351:dbl[])
        n153 = Bundle(w351, w353) -> (w359:cluster{dbl[], dbl[]})  [unwired: 1 in]
        n154 = Bundle(w351, w352) -> (w360:cluster{dbl[], dbl[]})  [unwired: 1 in]
        n155 = Build Array(w359, w360) -> (w348:cluster{dbl[], dbl[]}[])
        n156 = call-poly <userlib>:"Linear Fit.vi"("XY-data"=w348) -> ("Best Fits"=w347:cluster{"X-array":dbl[], "Y-array":dbl[]}[], "XY-data out"=w346:cluster{"X-array":dbl[], "Y-array":dbl[]}[], "slopes"=w345:dbl[])  [unwired: 4 in, 4 out]
        n157 = Multiply(x=w345, y=8.617333e-05) -> (x*y=→"E_a":dbl[])
        n158 = Interleave 1D Arrays(w346, w347) -> (→"Arrhenius":cluster{"X-array":dbl[], "Y-array":dbl[]}[])
        n159 = call <vilib>:"Add State(s) to Queue__jki_lib_state_machine.vi"("State(s) in (\"\")"=w372) -> ("States Out"=w371:string)  [unwired: 14 in]
      }
      frame "Analysis: Lifespan" {
        w383 = 3600
        # "Template Separator\n(You can make a copy of, or modify, this frame)"
        n160 = Unbundle By Name(w396) -> ("G2T 1D"=w407:cluster{dbl[], dbl[]}[], "G4T 1D"=w406:cluster{dbl[], dbl[]}[], "Final Temp"=w403:i32, "Init Temp"=w395:i32, "Temp Step"=w394:i32)  [unwired: 3 out]
        n161 = Subtract(x=w403, y=w395) -> (x-y=w404:i32)
        n162 = Divide(x=w404, y=w394) -> (x/y=w405:dbl)
        n163 = Increment(x=w405) -> (x+1=w393:dbl)
        n164 = for {
          N: w393 -> [_]
          tunnel: w395 -> [w419]
          tunnel: w394 -> [w418]
          tunnel: [w417] -> w392 mode=indexing
          i -> [w420]
          n165 = Multiply(x=w418, y=w420) -> (x*y=w421:i32)
          n166 = Add(x=w419, y=w421) -> (x+y=w417:i32)
        }
        n167 = call <userlib>:"Linear Fit (multiple).vi"("XY-data"=w407) -> ("XY-data out"=w389:cluster{"X-array":dbl[], "Y-array":dbl[]}[], "slopes"=w391:dbl[])  [unwired: 4 in, 5 out]
        n168 = call <userlib>:"Linear Fit (multiple).vi"("XY-data"=w406) -> ("XY-data out"=w388:cluster{"X-array":dbl[], "Y-array":dbl[]}[], "slopes"=w390:dbl[])  [unwired: 4 in, 5 out]
        n169 = for {
          tunnel: w389 -> [w415] mode=indexing
          tunnel: w388 -> [w416] mode=indexing
          tunnel: [w412] -> w387 mode=indexing
          tunnel: [w411] -> w386 mode=indexing
          n170 = Unbundle(w415) -> ("Y-array"=w413:dbl[])  [unwired: 1 out]
          n171 = Unbundle(w416) -> ("Y-array"=w414:dbl[])  [unwired: 1 out]
          n172 = call-poly <vilib>:"Mean.vi"("X"=w414) -> ("mean"=w411:dbl)  [unwired: 1 out]
          n173 = call-poly <vilib>:"Mean.vi"("X"=w413) -> ("mean"=w412:dbl)  [unwired: 1 out]
        }
        n174 = Divide(x=w387, y=w391) -> (x/y=w385:dbl[])
        n175 = Divide(x=w386, y=w390) -> (x/y=w384:dbl[])
        n176 = Divide(x=w385, y=w383) -> (x/y=w381:dbl[])
        n177 = Divide(x=w384, y=w383) -> (x/y=w382:dbl[])
        n178 = Array Subset(array=w381, length="Temps to keep (Lifespan)") -> (w399:dbl[])  [unwired: 1 in]
        n179 = Array Subset(array=w382, length="Temps to keep (Lifespan)") -> (w398:dbl[])  [unwired: 1 in]
        n180 = Array Subset(array=w392, length="Temps to keep (Lifespan)") -> (w397:i32[])  [unwired: 1 in]
        n181 = Absolute Value(x=w399) -> (abs(x)=w379:dbl[])
        n182 = Absolute Value(x=w398) -> (abs(x)=w380:dbl[])
        n183 = Bundle(w397, w379) -> (w401:cluster{i32[], dbl[]})  [unwired: 1 in]
        n184 = Bundle(w397, w380) -> (w402:cluster{i32[], dbl[]})  [unwired: 1 in]
        n185 = Build Array(w401, w402) -> ()  [unwired: 1 out]
        n186 = call <vilib>:"Add State(s) to Queue__jki_lib_state_machine.vi"("State(s) in (\"\")"=w410) -> ("States Out"=w409:string)  [unwired: 14 in]
      }
    }
  }
  "error out" <- w1
